vi "pci-6713-6025E-6733(set all analog)_update.vi"(4 "6221 Control":dbl[](array[numeric])=[6.5, 7.0], 5 "Change 6221?":bool, 6 "6733 Control":sgl[](array[numeric])=[8.0, 3.0, 4.0, 0.0, 0.0, 6.46, 6.98, 0.0] format="%.3f", 7 "Change 6733":bool, 8 "6713 Control":sgl[](array[numeric])=[4.6, 0.5, 0.035, 7.35, 10.0, 4.0, 4.0, 2.703] format="%.3f", 9 "Change 6713?":bool=TRUE) -> (0 "Voltage limit (+-10V)":string[](array[string])=["OK ", "OK ", "OK ", "OK ", "OK ", "OK ", "OK ", "OK "], 1 "6733 Status":string="PCI-6733 OK", 2 "Voltage limit (+-10V)":string[](array[string])=["OK ", "OK ", "OK ", "OK ", "OK ", "OK ", "OK ", "OK "], 3 "6713 Status":string="PCI-6713 OK")   [LabVIEW 2013]
uses:
  <vilib>/DAQmx/write.llb/DAQmx Write (Analog DBL 1Chan 1Samp).vi
  <vilib>/DAQmx/create/channels.llb/DAQmx Create Channel (AO-Voltage-Basic).vi
  <vilib>/DAQmx/miscellaneous.llb/DAQmx Fill In Error Info.vi
  pci-6713-6025E-6733(set all analog).vi/AO Update Channel (scaled value).vi
  Instance           4 43Saved   pci-6713-6025E-6733(set all analog) .vi
  Instance           5 43Saved   pci-6713-6025E-6733(set all analog) .vi
  <resource>/objmgr/daqmx.rc
panel:
  out "DAQmx Device Name":tag
  in  "Case Constant\n(See Context Help) 4":bool
  in  "Case Constant\n(See Context Help) 3":bool
  in  "Case Constant\n(See Context Help) 2":bool
  in  "Change 6025?":bool
  in  "Case Constant\n(See Context Help)":bool
  out "6733 Status 2":string="PCI-6733 OK"
  in  "6733 Control 2":sgl[](array[numeric])=[8.0, 3.0, 4.0, 0.0, 0.0, 6.46, 6.98, 0.0] format="%.3f"
  out "Voltage limit (+-10V) 2":string[](array[string])=["OK ", "OK ", "OK ", "OK ", "OK ", "OK ", "OK ", "OK "]
  out "Array 3":sgl[](array[numeric])=[8.0, 3.0, 4.0, 0.0, 0.0, 6.46, 6.98, 0.0]
  out "error out":errorcluster
  in  "Change 87Sr 6733":bool
  in  "87Sr 6733 Control":sgl[](array[numeric])=[8.0, 3.0, 4.0, 0.0, 0.0, 6.46, 6.98, 0.0] format="%.3f"
  out "87Sr Voltage limit (+-10V)":string[](array[string])=["OK ", "OK ", "OK ", "OK ", "OK ", "OK ", "OK ", "OK "]
  out "Array 2":sgl[](array[numeric])=[8.0, 3.0, 4.0, 0.0, 0.0, 6.46, 6.98, 0.0]
  out "Array":sgl[](array[numeric])=[8.0, 3.0, 4.0, 0.0, 0.0, 6.46, 6.98, 0.0]
  out "Voltage Limit (":string[](array[string])=["OK ", "OK "]
  in  "6025 Control":sgl[](array[numeric])=[-0.15, 0.1] format="%.3f"
  out "6025 Status":string="PCI-6025E OK"
  # "0..satabs offset for imaging"
  # "1... MOT power"
  # "2....MOT Jump Power"
  # "3....GENERAL PARAMETER: PAS AOM"
  # "4... GenPAram: offset lock"
  # "5....Vset for Lambda (0 to 10V)(pos for FET lock)"
  # "The DC supply\nvoltage for the\nZOS was 14.1 V"
  # "6....satabs offset for MOT"
  # "7.... satabs offset for cooling"
  # "0.....422 image AOM"
  # "PCI-6025E is NOT functional for Neutral Atoms.\nIt has been disabled in the block diagram, so\nchanging any of these values will not affect \nanything."
  # "1.....openr"
  # "Right now, put in units of \nvolts.  Freq to voltage \nconversion later."
  # "0.....100MHz Red MOT AOM (ZOS100) MHZ"
  # "1..... Power Control on  Red MOT AOM 5V full"
  # "dimage1 6.46V = 51.81MHz"
  # "dmot 6.980V = 35.50MHz"
  # "0.. Image AOM VCO (5V=41.5)"
  # "0..MOT AOM VCO (5V=41.5)"
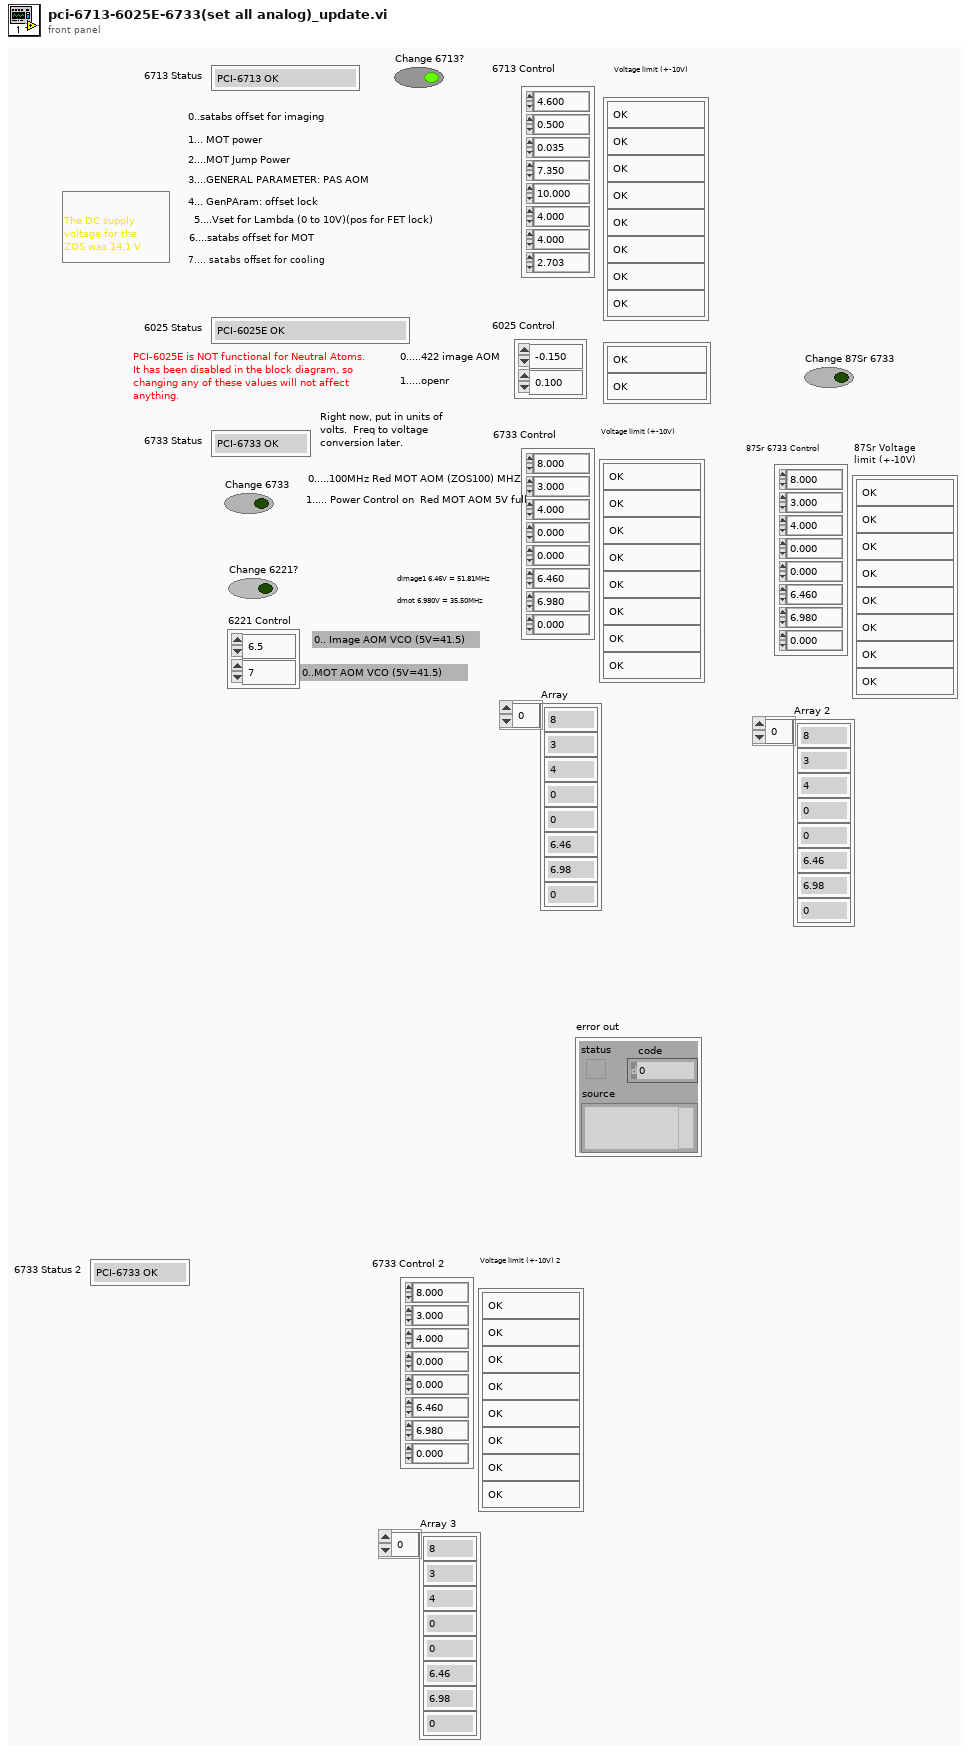
[diagram p1: front panel]
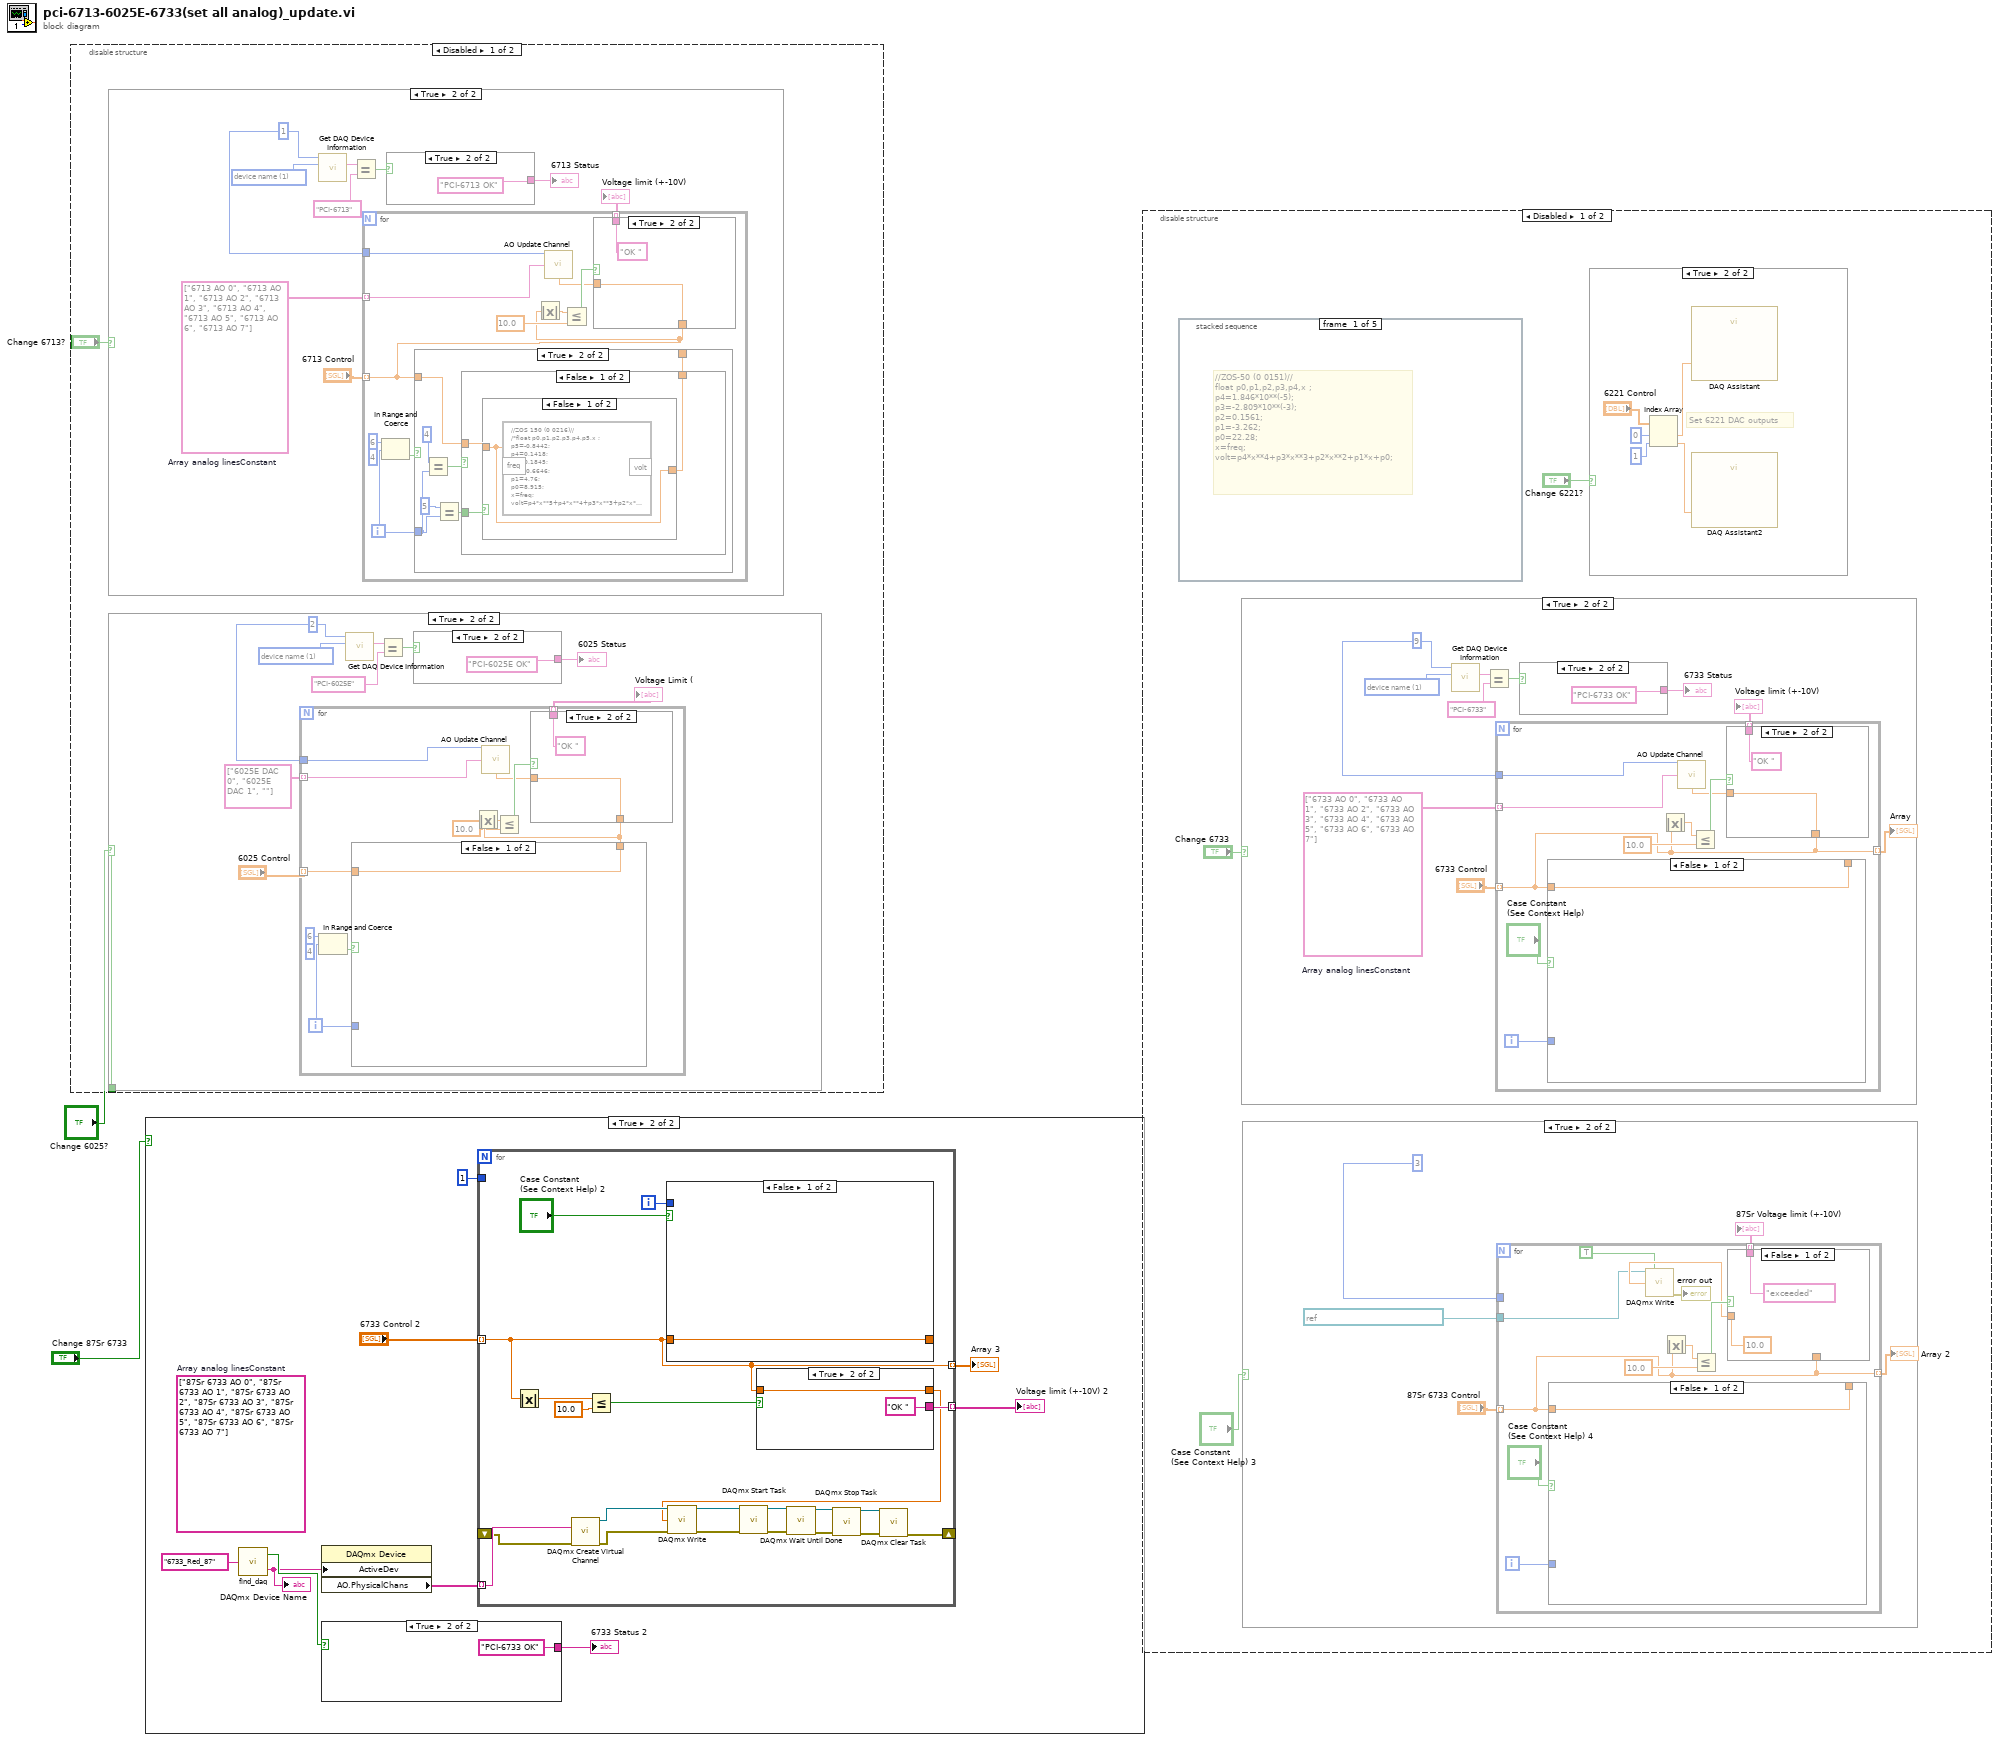
[diagram p0: block diagram]
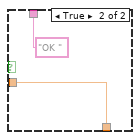
[diagram p3: hidden frame]
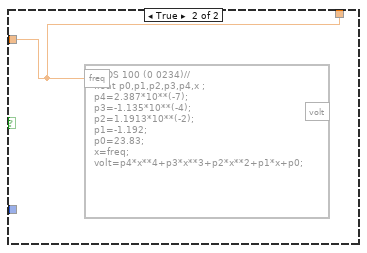
[diagram p4: hidden frame]
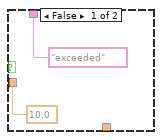
[diagram p7: hidden frame]
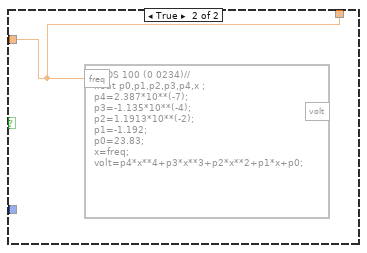
[diagram p8: hidden frame]
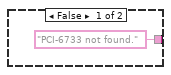
[diagram p9: hidden frame]
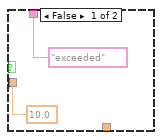
[diagram p16: hidden frame]
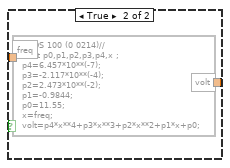
[diagram p18: hidden frame]
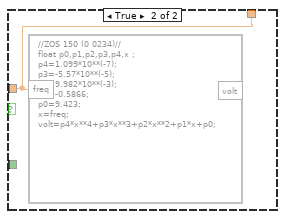
[diagram p19: hidden frame]
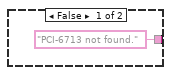
[diagram p20: hidden frame]
diagram:
  n1 = disable-structure shown="Disabled" {
    disable-tunnel: "Change 6025?" -> [w3 _]
    frame Disabled {
      n2 = case shown="True" "Change 6713?" {
        frame False {
        }
        frame True {
          w5 = tag[] ["6713 AO 0", "6713 AO 1", "6713 AO 2", "6713 AO 3", "6713 AO 4", "6713 AO 5", "6713 AO 6", "6713 AO 7"]  # Array analog linesConstant
          w13 = u32 1 items=["NI-DAQ version", "device name", "base address", "data transfer mode for analog input", "data transfer mode for analog output group 1", "data transfer mode for analog output group 2", "data transfer mode for GPCTR 0", "data transfer mode for GPCTR 1", "data transfer mode for digital I/O group 1", "data transfer mode for digital I/O group 2", "device type code", "DMA A level", "DMA B level", "DMA C level", "interrupt A level", "interrupt B level", "reserved", "lpt device mode", "DAQCard-700 counter 1 source", "interrupt generation mode", "device state during suspend mode", "computer name", "serial number", "counter type"] ("information type")
          w8 = u32 1 ("task ID or device")
          n3 = call "Get DAQ Device Information.vi"("information type"=w13, "task ID or device"=w8) -> ("information string"=w12:string)  [unwired: 7 in, 2 out]
          n4 = Equal?(x=w12, y="PCI-6713") -> (x = y?=w10:bool)
          n5 = for {
            tunnel: w8 -> [w25]
            tunnel: "6713 Control" -> [w14] mode=indexing
            tunnel: w5 -> [w24] mode=indexing
            tunnel: [w15] -> w6 mode=indexing
            i -> [w23]
            n6 = In Range and Coerce(upper limit=6, x=w23, lower limit=4) -> (In Range?=w20:bool)  [unwired: 1 out]
            n7 = case shown="True" w20 {
              tunnel: w14 -> [w30 w32]
              tunnel: [w30 w31] -> _
              tunnel: w23 -> [_ w35]
              frame False {
              }
              frame True {
                n8 = Equal?(x=4, y=w35) -> (x = y?=w36:bool)
                n9 = Equal?(x=5, y=w35) -> (x = y?=w33:bool)
                n10 = case shown="False" w36 {
                  tunnel: w33 -> [w40 _]
                  tunnel: w32 -> [w39 w44]
                  tunnel: [w38 w44] -> w31
                  frame False {
                    n11 = case shown="False" w40 {
                      tunnel: w39 -> [w41 w43]
                      tunnel: [w41 w42] -> w38
                      frame False {
                        n12 = formula code="//ZOS 150 (0 0216)//\n/*float p0,p1,p2,p3,p4,p5,x ;\np5=-0.8442;\np4=0.1418;\np3=0.1845;\np2=-0.6646;\np1=4.76;\np0=8.915;\nx=freq;\nvolt=p4*x**5+p4*x**4+p3*x**3+p2*x**2+p1*x+p0;\n*/\nvolt=freq;"("freq"=w41) -> ()  [unwired: 1 out]
                      }
                      frame True {
                        n13 = formula code="//ZOS 100 (0 0214)//\nfloat p0,p1,p2,p3,p4,x ;\np4=6.457*10**(-7);\np3=-2.117*10**(-4);\np2=2.473*10**(-2);\np1=-0.9844;\np0=11.55;\nx=freq;\nvolt=p4*x**4+p3*x**3+p2*x**2+p1*x+p0;"("freq"=w43) -> ("volt"=w42:dbl)
                      }
                    }
                  }
                  frame True {
                    n14 = formula code="//ZOS 150 (0 0234)//\nfloat p0,p1,p2,p3,p4,x ;\np4=1.099*10**(-7);\np3=-5.57*10**(-5);\np2=9.982*10**(-3);\np1=-0.5866;\np0=9.423;\nx=freq;\nvolt=p4*x**4+p3*x**3+p2*x**2+p1*x+p0;"("freq"=w44) -> ()  [unwired: 1 out]
                  }
                }
              }
            }
            n15 = Absolute Value(x=w14) -> (abs(x)=w19:sgl)
            n16 = Less Or Equal?(x=w19, y=10.0) -> (x <= y?=w17:bool)
            n17 = case shown="True" w17 {
              tunnel: w14 -> [_ w29]
              tunnel: [10.0 w29] -> w16
              tunnel: ["exceeded" ("String") "OK " ("String")] -> w15
              frame False {
              }
              frame True {
              }
            }
            n18 = call-poly "AO Update Channel.vi"("value"=w16, "channel (0)"=w24, "device"=w25) -> ()
          }
          "Voltage limit (+-10V)" <- w6
          n19 = case shown="True" w10 {
            tunnel: ["PCI-6713 not found." "PCI-6713 OK"] -> w9
            frame False {
            }
            frame True {
            }
          }
          "6713 Status" <- w9
        }
      }
      n20 = case shown="True" w3 {
        frame False {
        }
        frame True {
          w55 = u32 1 items=["NI-DAQ version", "device name", "base address", "data transfer mode for analog input", "data transfer mode for analog output group 1", "data transfer mode for analog output group 2", "data transfer mode for GPCTR 0", "data transfer mode for GPCTR 1", "data transfer mode for digital I/O group 1", "data transfer mode for digital I/O group 2", "device type code", "DMA A level", "DMA B level", "DMA C level", "interrupt A level", "interrupt B level", "reserved", "lpt device mode", "DAQCard-700 counter 1 source", "interrupt generation mode", "device state during suspend mode", "computer name", "serial number", "counter type"] ("information type")
          w50 = u32 2 ("task ID or device")
          n21 = for {
            tunnel: w50 -> [w68]
            tunnel: "6025 Control" -> [w62] mode=indexing
            tunnel: tag[] ["6025E DAC 0", "6025E DAC 1", ""] ("Array analog linesConstant") -> [w67] mode=indexing
            tunnel: [w56] -> w48 mode=indexing
            i -> [w66]
            n22 = In Range and Coerce(upper limit=6, x=w66, lower limit=4) -> (In Range?=w63:bool)  [unwired: 1 out]
            n23 = case shown="False" w63 {
              tunnel: w62 -> [w73 w75]
              tunnel: [w73 w74] -> w61
              tunnel: w66 -> [_ w78]
              frame False {
              }
              frame True {
                n24 = Equal?(x=4, y=w78) -> (x = y?=w79:bool)
                n25 = Equal?(x=5, y=w78) -> (x = y?=w76:bool)
                n26 = case shown="False" w79 {
                  tunnel: w76 -> [w83 _]
                  tunnel: w75 -> [w82 w89]
                  tunnel: [w81 w88] -> w74
                  frame False {
                    n27 = case shown="False" w83 {
                      tunnel: w82 -> [w85 w87]
                      tunnel: [w84 w86] -> w81
                      frame False {
                        n28 = formula code="//ZOS 150 (0 0234)//\n/*float p0,p1,p2,p3,p4,x ;\np4=1.099*10**(-7);\np3=-5.57*10**(-5);\np2=9.982*10**(-3);\np1=-0.5856;\np0=9.423;\nx=freq;\nvolt=p4*x**4+p3*x**3+p2*x**2+p1*x+p0-3\n;*/\nvolt=freq;"("freq"=w85) -> ("volt"=w84:dbl)
                      }
                      frame True {
                        n29 = formula code="//ZOS-50 (0 0151)//\nfloat p0,p1,p2,p3,p4,x ;\np4=1.846*10**(-5);\np3=-2.809*10**(-3);\np2=0.1561;\np1=-3.262;\np0=22.28;\nx=freq;\nvolt=p4*x**4+p3*x**3+p2*x**2+p1*x+p0;"("freq"=w87) -> ("volt"=w86:dbl)
                      }
                    }
                  }
                  frame True {
                    n30 = formula code="//ZOS 50 (0 0233)//\nfloat p0,p1,p2,p3,p4,x ;\np4=3.992*10**(-6);\np3=-6.824*10**(-4);\np2=4.095*10**(-2);\np1=-0.5384;\np0=-1.048;\nx=freq;\nvolt=p4*x**4+p3*x**3+p2*x**2+p1*x+p0;"("freq"=w89) -> ("volt"=w88:dbl)
                  }
                }
              }
            }
            n31 = Absolute Value(x=w61) -> (abs(x)=w60:dbl)
            n32 = Less Or Equal?(x=w60, y=10.0) -> (x <= y?=w58:bool)
            n33 = case shown="True" w58 {
              tunnel: w61 -> [_ w72]
              tunnel: [10.0 w72] -> w57
              tunnel: ["exceeded" ("String") "OK " ("String")] -> w56
              frame False {
              }
              frame True {
              }
            }
            n34 = call-poly "AO Update Channel.vi"("value"=w57, "channel (0)"=w67, "device"=w68) -> ()
          }
          "Voltage Limit (" <- w48
          n35 = call "Get DAQ Device Information.vi"("information type"=w55, "task ID or device"=w50) -> ("information string"=w54:string)  [unwired: 7 in, 2 out]
          n36 = Equal?(x=w54, y="PCI-6025E") -> (x = y?=w52:bool)
          n37 = case shown="True" w52 {
            tunnel: ["PCI-6025E not found." "PCI-6025E OK"] -> w51
            frame False {
            }
            frame True {
            }
          }
          "6025 Status" <- w51
        }
      }
    }
    frame Enabled {
    }
  }
  n38 = case shown="True" "Change 87Sr 6733" {
    frame False {
    }
    frame True {
      (unwired) tag[] ["87Sr 6733 AO 0", "87Sr 6733 AO 1", "87Sr 6733 AO 2", "87Sr 6733 AO 3", "87Sr 6733 AO 4", "87Sr 6733 AO 5", "87Sr 6733 AO 6", "87Sr 6733 AO 7"]  # Array analog linesConstant
      n39 = call "find_daq.vi"("Device Name"="6733_Red_87") -> ("Device Present"=w95:bool, "DAQmx Device Name"=w93:tag)
      "DAQmx Device Name" <- w93
      n40 = property class="DAQmx Device"("ActiveDev"=w93) -> ("AO.PhysicalChans"=w92:tag[])  [unwired: 2 in, 2 out]
      n41 = case shown="True" w95 {
        tunnel: ["PCI-6733 not found." "PCI-6733 OK"] -> w100
        frame False {
        }
        frame True {
        }
      }
      "6733 Status 2" <- w100
      n42 = for {
        tunnel: u32 1 ("task ID or device") -> [_]
        tunnel: "6733 Control 2" -> [w115] mode=indexing
        tunnel: w92 -> [w114] mode=indexing
        tunnel: [w118] -> w97 mode=indexing
        tunnel: [w115] -> w96 mode=indexing
        shift-right: [w102] -> _
        shift-left: _ -> [w101]
        i -> [w117]
        n43 = Absolute Value(x=w115) -> (abs(x)=w121:sgl)
        n44 = call-poly <vilib>:"DAQmx Create Virtual Channel.vi"("physical channels"=w114, "error in"=w101) -> ("task out"=w113:refnum<k21>, "error out"=w111:errorcluster)  [unwired: 12 in]
        n45 = Less Or Equal?(x=w121, y=10.0) -> (x <= y?=w119:bool)
        n46 = case shown="False" "Case Constant\n(See Context Help) 2" {
          tunnel: w115 -> [w126 w127]
          tunnel: [w126 w127] -> _
          tunnel: w117 -> [_ _]
          frame False {
          }
          frame True {
            n47 = formula code="//ZOS 100 (0 0234)//\nfloat p0,p1,p2,p3,p4,x ;\np4=2.387*10**(-7);\np3=-1.135*10**(-4);\np2=1.1913*10**(-2);\np1=-1.192;\np0=23.83;\nx=freq;\nvolt=p4*x**4+p3*x**3+p2*x**2+p1*x+p0;"("freq"=w127) -> ()  [unwired: 1 out]
          }
        }
        n48 = case shown="True" w119 {
          tunnel: w115 -> [_ w125]
          tunnel: [10.0 w125] -> w112
          tunnel: ["exceeded" ("String") "OK " ("String")] -> w118
          frame False {
          }
          frame True {
          }
        }
        n49 = call-poly <vilib>:"DAQmx Write.vi"("task/channels in"=w113, "data"=w112, "error in"=w111) -> ("task out"=w109:refnum<k21>, "error out"=w110:errorcluster)  [unwired: 10 in, 1 out]
        n50 = call <vilib>:"DAQmx Start Task.vi"("task/channels in"=w109, "error in"=w110) -> ("task out"=w108:refnum<k21>, "error out"=w107:errorcluster)  [unwired: 12 in]
        n51 = call <vilib>:"DAQmx Wait Until Done.vi"("task/channels in"=w108, "error in"=w107) -> ("task out"=w106:refnum<k21>, "error out"=w105:errorcluster)  [unwired: 12 in]
        n52 = call <vilib>:"DAQmx Stop Task.vi"("task/channels in"=w106, "error in"=w105) -> ("task out"=w104:refnum<k21>, "error out"=w103:errorcluster)  [unwired: 12 in]
        n53 = call <vilib>:"DAQmx Clear Task.vi"("task in"=w104, "error in"=w103) -> ("error out"=w102:errorcluster)  [unwired: 13 in]
      }
      "Voltage limit (+-10V) 2" <- w97
      "Array 3" <- w96
    }
  }
  n54 = disable-structure shown="Disabled" {
    frame Disabled {
      n55 = stacked-sequence {
        frame #0 {
          # "//ZOS-50 (0 0151)//\nfloat p0,p1,p2,p3,p4,x ;\np4=1.846*10**(-5);\np3=-2.809*10**(-3);\np2=0.1561;\np1=-3.262;\np0=22.28;\nx=freq;\nvolt=p4*x**4+p3*x**3+p2*x**2+p1*x+p0;"
        }
        frame #1 {
          # "//ZOS 100 (0 0214)//\nfloat p0,p1,p2,p3,p4,x ;\np4=6.457*10**(-7);\np3=-2.117*10**(-4);\np2=2.473*10**(-2);\np1=-0.9844;\np0=11.55;\nx=freq;\nvolt=p4*x**4+p3*x**3+p2*x**2+p1*x+p0;"
        }
        frame #2 {
          # "//ZOS 150 (0 0234)//\nfloat p0,p1,p2,p3,p4,x ;\np4=1.099*10**(-7);\np3=-5.57*10**(-5);\np2=9.982*10**(-3);\np1=-0.5866;\np0=9.423;\nx=freq;\nvolt=p4*x**4+p3*x**3+p2*x**2+p1*x+p0;"
        }
        frame #3 {
          # "//ZOS 50 (0 0233)//\nfloat p0,p1,p2,p3,p4,x ;\np4=3.992*10**(-6);\np3=-6.824*10**(-4);\np2=4.095*10**(-2);\np1=-0.5384;\np0=-1.048;\nx=freq;\nvolt=p4*x**4+p3*x**3+p2*x**2+p1*x+p0;"
        }
        frame #4 {
          # "//ZOS 150 (0 0216)//\nfloat p0,p1,p2,p3,p4,p5,x ;\np5=-0.8442\np4=0.1418;\np3=0.1845;\np2=-0.6646;\np1=4.76;\np0=8.915;\nx=freq;\nvolt=p4*x**5+p4*x**4+p3*x**3+p2*x**2+p1*x+p0;"
        }
      }
      n56 = case shown="True" "Change 6733" {
        frame False {
        }
        frame True {
          w161 = tag[] ["6733 AO 0", "6733 AO 1", "6733 AO 2", "6733 AO 3", "6733 AO 4", "6733 AO 5", "6733 AO 6", "6733 AO 7"]  # Array analog linesConstant
          w169 = u32 1 items=["NI-DAQ version", "device name", "base address", "data transfer mode for analog input", "data transfer mode for analog output group 1", "data transfer mode for analog output group 2", "data transfer mode for GPCTR 0", "data transfer mode for GPCTR 1", "data transfer mode for digital I/O group 1", "data transfer mode for digital I/O group 2", "device type code", "DMA A level", "DMA B level", "DMA C level", "interrupt A level", "interrupt B level", "reserved", "lpt device mode", "DAQCard-700 counter 1 source", "interrupt generation mode", "device state during suspend mode", "computer name", "serial number", "counter type"] ("information type")
          w164 = u32 9 ("task ID or device")
          n57 = call "Get DAQ Device Information.vi"("information type"=w169, "task ID or device"=w164) -> ("information string"=w168:string)  [unwired: 7 in, 2 out]
          n58 = Equal?(x=w168, y="PCI-6733") -> (x = y?=w166:bool)
          n59 = for {
            tunnel: w164 -> [w179]
            tunnel: "6733 Control" -> [w170] mode=indexing
            tunnel: w161 -> [w178] mode=indexing
            tunnel: [w173] -> w162 mode=indexing
            tunnel: [w170] -> w160 mode=indexing
            i -> [w172]
            n60 = case shown="False" "Case Constant\n(See Context Help)" {
              tunnel: w170 -> [w184 w185]
              tunnel: [w184 w185] -> _
              tunnel: w172 -> [_ _]
              frame False {
              }
              frame True {
                n61 = formula code="//ZOS 100 (0 0234)//\nfloat p0,p1,p2,p3,p4,x ;\np4=2.387*10**(-7);\np3=-1.135*10**(-4);\np2=1.1913*10**(-2);\np1=-1.192;\np0=23.83;\nx=freq;\nvolt=p4*x**4+p3*x**3+p2*x**2+p1*x+p0;"("freq"=w185) -> ()  [unwired: 1 out]
              }
            }
            n62 = Absolute Value(x=w170) -> (abs(x)=w177:sgl)
            n63 = Less Or Equal?(x=w177, y=10.0) -> (x <= y?=w175:bool)
            n64 = case shown="True" w175 {
              tunnel: w170 -> [_ w183]
              tunnel: [10.0 w183] -> w174
              tunnel: ["exceeded" ("String") "OK " ("String")] -> w173
              frame False {
              }
              frame True {
              }
            }
            n65 = call-poly "AO Update Channel.vi"("value"=w174, "channel (0)"=w178, "device"=w179) -> ()
          }
          "Voltage limit (+-10V)" <- w162
          "Array" <- w160
          n66 = case shown="True" w166 {
            tunnel: ["PCI-6733 not found." "PCI-6733 OK"] -> w165
            frame False {
            }
            frame True {
            }
          }
          "6733 Status" <- w165
        }
      }
      n67 = case shown="True" "Case Constant\n(See Context Help) 3" {
        frame False {
        }
        frame True {
          n68 = for {
            tunnel: u32 3 ("task ID or device") -> [_]
            tunnel: "87Sr 6733 Control" -> [w142] mode=indexing
            tunnel: [w145] -> w135 mode=indexing
            tunnel: [w142] -> w134 mode=indexing
            tunnel: refnum<k21> "Red MOT Arbitrary Waveform Sr87" ("task/channels in") -> [w140]
            i -> [w144]
            n69 = case shown="False" "Case Constant\n(See Context Help) 4" {
              tunnel: w142 -> [w153 w154]
              tunnel: [w153 w154] -> _
              tunnel: w144 -> [_ _]
              frame False {
              }
              frame True {
                n70 = formula code="//ZOS 100 (0 0234)//\nfloat p0,p1,p2,p3,p4,x ;\np4=2.387*10**(-7);\np3=-1.135*10**(-4);\np2=1.1913*10**(-2);\np1=-1.192;\np0=23.83;\nx=freq;\nvolt=p4*x**4+p3*x**3+p2*x**2+p1*x+p0;"("freq"=w154) -> ()  [unwired: 1 out]
              }
            }
            n71 = Absolute Value(x=w142) -> (abs(x)=w148:sgl)
            n72 = Less Or Equal?(x=w148, y=10.0) -> (x <= y?=w146:bool)
            n73 = case shown="False" w146 {
              tunnel: w142 -> [_ w152]
              tunnel: [10.0 w152] -> w141
              tunnel: ["exceeded" ("String") "OK " ("String")] -> w145
              frame False {
              }
              frame True {
              }
            }
            n74 = call-poly <vilib>:"DAQmx Write.vi"("task/channels in"=w140, "auto start"=TRUE, "data"=w141) -> ("error out"=→"error out":errorcluster)  [unwired: 10 in, 2 out]
          }
          "87Sr Voltage limit (+-10V)" <- w135
          "Array 2" <- w134
        }
      }
      n75 = case shown="True" "Change 6221?" {
        frame False {
        }
        frame True {
          # "Set 6221 DAC outputs"
          n76 = Index Array(array="6221 Control", index #1=0 ("index"), index #2=1 ("index")) -> (element #1=w156:dbl, element #2=w155:dbl)
          n77 = call "DAQ Assistant"("data"=w156) -> ()  [unwired: 9 in, 2 out]
          n78 = call "DAQ Assistant2"("data"=w155) -> ()  [unwired: 9 in, 2 out]
        }
      }
    }
    frame Enabled {
    }
  }
